vi "Handle RESULT.vi"(8 "error in (no error)":errorcluster, 9 "Message Loop Shift Register Data":T1, 10 "WAMP Message":T16 {"Message Codes" items=["HELLO"=1, "WELCOME"=2, "ABORT"=3, "GOODBYE"=6, "ERROR"=8, "PUBLISH"=16, "PUBLISHED"=17, "SUBSCRIBE"=32, "SUBSCRIBED"=33, "UNSUBSCRIBE"=34, "UNSUBSCRIBED"=35, "EVENT"=36, "CALL"=48, "RESULT"=59, "REGISTER"=64, "REGISTERED"=65, "UNREGISTER"=66, "UNREGISTERED"=67, "INVOCATION"=68, "YIELD"=70]}, 11 "reference":refnum<class "WAMP Client.lvclass">) -> (0 "error out":errorcluster, 1 "Message Loop Shift Register Data (out)":T1, 3 "reference out":refnum<class "WAMP Client.lvclass">)   [LabVIEW 2020, in "wamplv.lvlib" / "WAMP Client.lvclass"]
uses:
  WAMP Client.lvclass
  TypeDef/WAMP Received Message.ctl
  TypeDef/WAMP Message Codes.ctl
  TypeDef/Message Loop Shift Reg Data.ctl
  TypeDef/REGISTER Request Data.ctl
  TypeDef/Success or error.ctl
  API/TypeDefs/Combined error.ctl
  API/TypeDefs/WAMP error.ctl
  TypeDef/Publish Requests Map.ctl
  TypeDef/PUBLISH Request Data.ctl
  TypeDef/PUBLISH result.ctl
  TypeDef/Endpoint Data.ctl
  TypeDef/CALL Request Map.ctl
  TypeDef/CALL Request Data.ctl
  API/TypeDefs/RESULT payload.ctl
  TypeDef/SUBSCRIBE Requests Map.ctl
  TypeDef/SUBSCRIBE Request Data.ctl
  TypeDef/Subscribe Result.ctl
  TypeDef/EVENT payload.ctl
  TypeDef/Subscriptions Map.ctl
  TypeDef/Subscription Details.ctl
  TypeDef/Unsubscribe Requests Map.ctl
  TypeDef/UNSUBSCRIBE Request Data.ctl
  TypeDef/UNSUBSCRIBE Result.ctl
  TypeDef/Unregister requests map.ctl
  TypeDef/Unregister request.ctl
  WAMP Client.lvclass/WAMP Client.ctl
  fe43fee3-e626-436a-9df9-4c595b512d78.vi
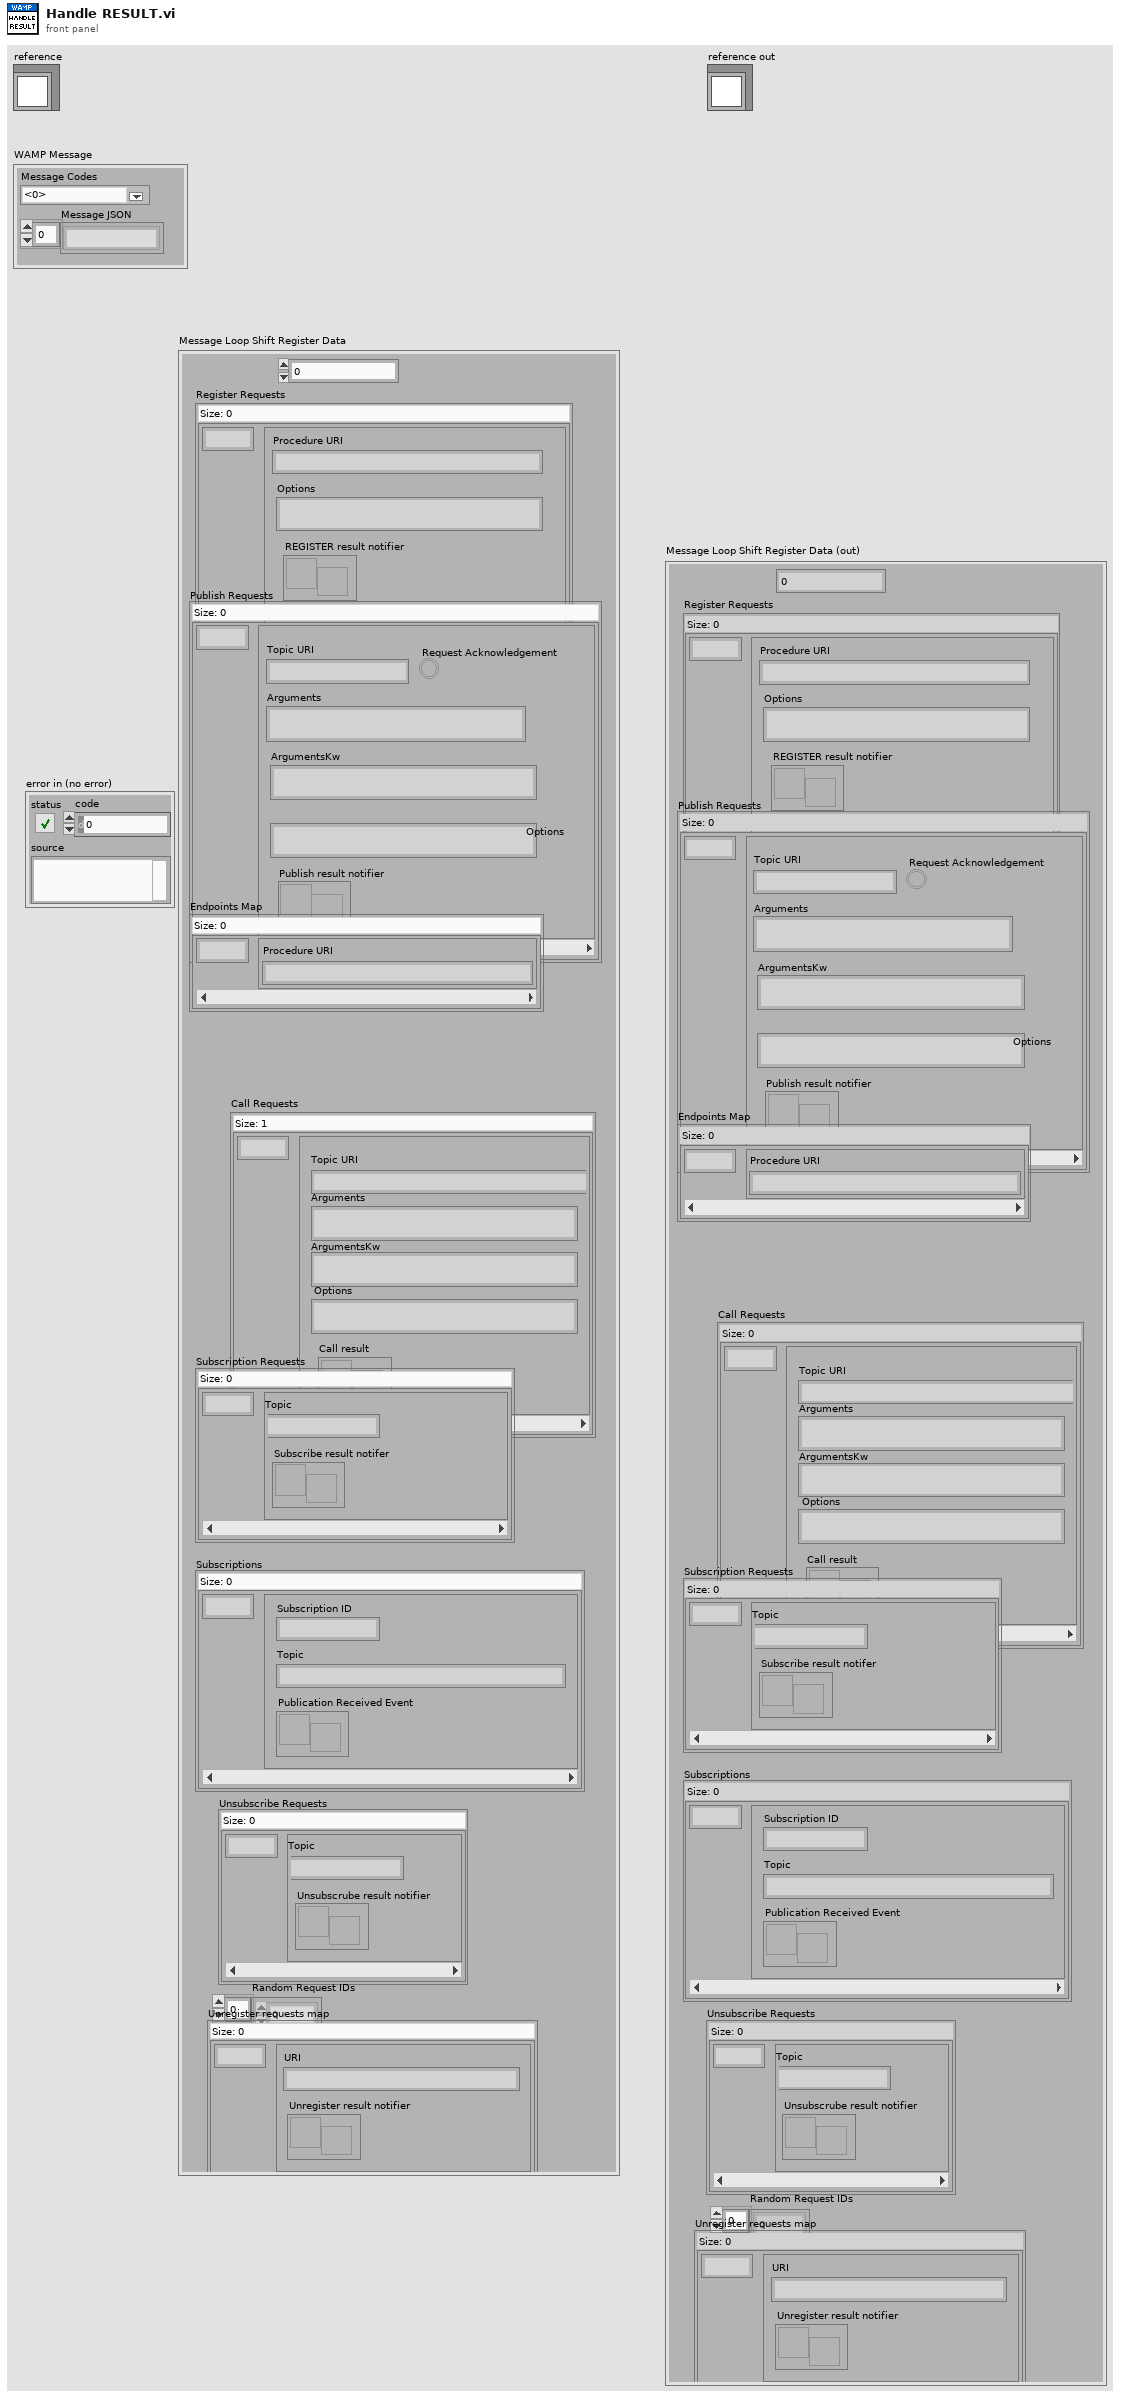
[diagram p1: front panel]
types:
  T1 = typedef "wamplv.lvlib/WAMP Client.lvclass/Message Loop Shift Reg Data.ctl" = cluster{"Last Request ID":u64, "Register Requests":map{u64, T2}, "Publish Requests":T3, "Endpoints Map":map{u64, T5}, "Call Requests":T6, "Subscription Requests":T8, "Subscriptions":T10, "Unsubscribe Requests":T12, "Random Request IDs":u64[], "Unregister requests map":T14}
  T2 = typedef "wamplv.lvlib/WAMP Client.lvclass/REGISTER Request Data.ctl" = cluster{"Procedure URI":string, "Options":string, "REGISTER result notifier":refnum<notifier>}
  T3 = typedef "wamplv.lvlib/WAMP Client.lvclass/Publish Requests Map.ctl" = map{u64, T4}
  T4 = typedef "wamplv.lvlib/WAMP Client.lvclass/PUBLISH Request Data.ctl" = cluster{"Topic URI":string, "Arguments":string, "ArgumentsKw":string, "Request Acknowledgement":bool, "Options":string, "Publish result notifier":refnum<notifier>}
  T5 = typedef "wamplv.lvlib/WAMP Client.lvclass/Endpoint Data.ctl" = cluster{"Procedure URI":string}
  T6 = typedef "wamplv.lvlib/WAMP Client.lvclass/CALL Request Map.ctl" = map{u64, T7}
  T7 = typedef "wamplv.lvlib/WAMP Client.lvclass/CALL Request Data.ctl" = cluster{"Topic URI":string, "Arguments":string, "ArgumentsKw":string, "Options":string, "Call result":refnum<notifier>}
  T8 = typedef "wamplv.lvlib/WAMP Client.lvclass/SUBSCRIBE Requests Map.ctl" = map{u64, T9}
  T9 = typedef "wamplv.lvlib/WAMP Client.lvclass/SUBSCRIBE Request Data.ctl" = cluster{"Topic":string, "Subscribe result notifer":refnum<notifier>}
  T10 = typedef "wamplv.lvlib/WAMP Client.lvclass/Subscriptions Map.ctl" = map{u64, T11}
  T11 = typedef "wamplv.lvlib/WAMP Client.lvclass/Subscription Details.ctl" = cluster{"Subscription ID":u64, "Topic":string, "Publication Received Event":refnum<user-event>}
  T12 = typedef "wamplv.lvlib/WAMP Client.lvclass/Unsubscribe Requests Map.ctl" = map{u64, T13}
  T13 = typedef "wamplv.lvlib/WAMP Client.lvclass/UNSUBSCRIBE Request Data.ctl" = cluster{"Topic":string, "Unsubscrube result notifier":refnum<notifier>}
  T14 = typedef "wamplv.lvlib/WAMP Client.lvclass/Unregister requests map.ctl" = map{u64, T15}
  T15 = typedef "wamplv.lvlib/WAMP Client.lvclass/Unregister request.ctl" = cluster{"URI":string, "Unregister result notifier":refnum<notifier>}
  T16 = typedef "wamplv.lvlib/WAMP Client.lvclass/WAMP Received Message.ctl" = cluster{"Message JSON":string[], "Message Codes":T17}
  T17 = typedef "wamplv.lvlib/WAMP Client.lvclass/WAMP Message Codes.ctl" = u16
  T18 = typedef "wamplv.lvlib/WAMP Client.lvclass/RESULT payload.ctl" = cluster{"Arguments Payload":string, "ArgumentKw Payload":string, "Topic":string, "Combined Error":T19}
  T19 = typedef "wamplv.lvlib/WAMP Client.lvclass/Combined error.ctl" = cluster{"Error?":bool, "WAMP Error":T20, "Error":errorcluster}
  T20 = typedef "wamplv.lvlib/WAMP Client.lvclass/WAMP error.ctl" = cluster{"Details":string, "ArgumentKw Payload":string, "Error?":bool, "Error URI":string, "Arguments Payload":string}
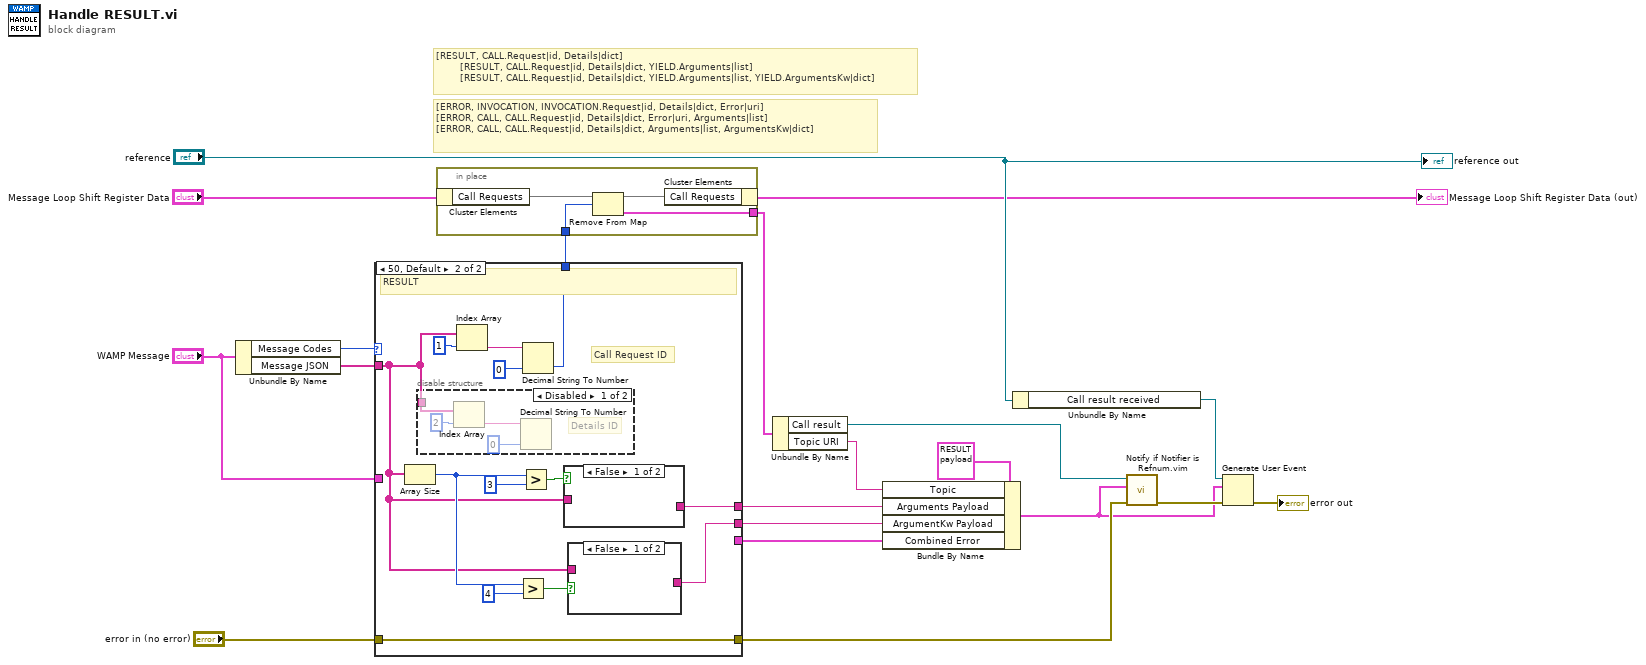
[diagram p0: block diagram]
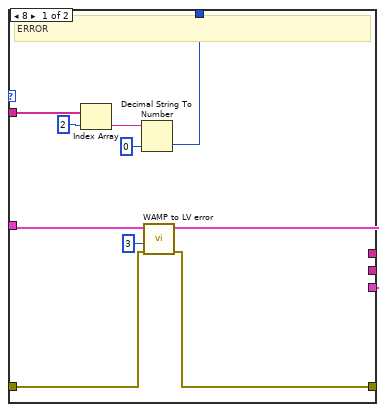
[diagram p2: hidden frame]
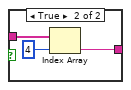
[diagram p4: hidden frame]
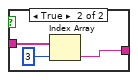
[diagram p5: hidden frame]
diagram:
  # "[ERROR, INVOCATION, INVOCATION.Request|id, Details|dict, Error|uri]\n[ERROR, CALL, CALL.Request|id, Details|dict, Error|uri, Arguments|list]\n[ERROR, CALL, CALL.Request|id, Details|dict, Arguments|list, ArgumentsKw|dict]"
  # "[RESULT, CALL.Request|id, Details|dict]\n        [RESULT, CALL.Request|id, Details|dict, YIELD.Arguments|list]\n        [RESULT, CALL.Request|id, Details|dict, YIELD.Arguments|list, YIELD.ArgumentsKw|dict]"
  n1 = Unbundle By Name("WAMP Message") -> ("Message Codes"=w19:T17, "Message JSON"=w18:string[])
  n2 = case shown="50, Default" w19 {
    tunnel: w18 -> [w27 w34]
    tunnel: [w28 w33] -> w17
    tunnel: "error in (no error)" -> [w22 w31]
    tunnel: [w21 w31] -> w7
    tunnel: [_ w36] -> w14
    tunnel: [_ w35] -> w13
    tunnel: [w24 _] -> w9
    tunnel: "WAMP Message" -> [w23 _]
    frame 8 {
      # "ERROR"
      n3 = Index Array(array=w27, index=2) -> (element=w29:string)
      n4 = Decimal String To Number(string=w29, default (0L)=u64 0 ("default (0 I32)")) -> (number=w28:u64)  [unwired: 1 in, 1 out]
      n5 = call "WAMP to LV error.vi"("error in (no error)"=w22, "Details Index"=u32 3, "WAMP Message"=w23) -> ("error out"=w21:errorcluster, "Combined Error"=w24:T19)  [unwired: 6 in, 1 out]
    }
    frame 50, Default {
      # "Call Request ID"
      # "RESULT"
      n6 = Array Size(array=w34) -> (size(s)=w37:i32)
      n7 = disable-structure shown="Disabled" {
        disable-tunnel: w34 -> [w44 _]
        frame Disabled {
          # "Details ID"
          n8 = Index Array(array=w44, index=2) -> (element=w47:string)
          n9 = Decimal String To Number(string=w47, default (0L)=u32 0) -> ()  [unwired: 1 in, 2 out]
        }
        frame Enabled {
        }
      }
      n10 = Index Array(array=w34, index=1) -> (element=w42:string)
      n11 = Greater?(x=w37, y=4) -> (0:w38:bool)
      n12 = Greater?(x=w37, y=3) -> (0:w32:bool)
      n13 = Decimal String To Number(string=w42, default (0L)=u64 0) -> (number=w33:u64)  [unwired: 1 in, 1 out]
      n14 = case shown="False" w32 {
        tunnel: [_ w51] -> w36
        tunnel: w34 -> [_ w52]
        frame False {
        }
        frame True {
          n15 = Index Array(array=w52, index=3) -> (element=w51:string)
        }
      }
      n16 = case shown="False" w38 {
        tunnel: [_ w49] -> w35
        tunnel: w34 -> [_ w48]
        frame False {
        }
        frame True {
          n17 = Index Array(array=w48, index=4) -> (element=w49:string)
        }
      }
    }
  }
  n18 = in-place "In Place Element Structure" {
    in-place-border: w17 -> [w57]
    in-place-border: [w56] -> w16
    n19 = in-place-cluster #1("Message Loop Shift Register Data") -> ("Call Requests"=w55:T6)
    n20 = Remove From Map(10:w57, 11:w55) -> (1:w56:T7, 3:w54:T6)  [unwired: 1 out]
    n21 = in-place-cluster #1("Call Requests"=w54) -> (→"Message Loop Shift Register Data (out)":T1)
  }
  n22 = Unbundle By Name(w16) -> ("Call result"=w6:refnum<notifier>, "Topic URI"=w2:string)
  n23 = Bundle By Name(cluster=T18 {"Arguments Payload"="", "ArgumentKw Payload"="", "Topic"="", "Combined Error"={"Error?"=FALSE, "WAMP Error"={"Details"="{}", "ArgumentKw Payload"="", "Error?"=FALSE, "Error URI"="", "Arguments Payload"=""}, "Error"={"status"=FALSE, "code"=0, "source"=""}}} ("RESULT Payload"), "Topic"=w2, "Arguments Payload"=w14, "ArgumentKw Payload"=w13, "Combined Error"=w9) -> (w5:T18)
  n24 = Unbundle By Name("reference") -> ("Call result received"=w11:refnum<user-event>)
  n25 = call "Notify if Notifier is Refnum.vim"("error in (no error)"=w7, "RESULT Payload"=w5, "Notifier in"=w6) -> ("error out"=w8:errorcluster)  [unwired: 8 in]
  n26 = Generate User Event(user event=w11, event data cluster=w5, error in=w8) -> (error out=→"error out":errorcluster)  [unwired: 1 in, 1 out]
  "reference out" <- "reference"
